vi "get information display strings.vi"(8 "error in":errorcluster, 11 "CEF_serializable node in":refnum<class "CEF_serializable node.lvclass">) -> (0 "error out":errorcluster, 1 "Data":string[](array[string]), 2 "Labels":string[](array[string]), 3 "CEF_serializable node out":refnum<class "CEF_serializable node.lvclass">)   [LabVIEW 2025, in "CEF.lvlib" / "CEF_serializable node.lvclass"]
doc: "Copyright 2017 National Instruments Corporation\n\nLicensed under the Apache License, Version 2.0 (the \"License\"); you may not use this file except in compliance with the License. You may obtain a copy of the License at http://www.apache.org/licenses/LICENSE-2.0\nUnless required by applicable law or agreed to in writing, software distributed under the License is distributed on an \"AS IS\" BASIS, WITHOUT WARRANTIES OR CONDITIONS OF ANY KIND, either express or implied. See the License for the specific language governing permissions and limitations under the License."
uses:
  CEF_serializable node.lvclass
  serializable configuration/CEF_serializable configuration.lvclass/CEF_serializable configuration.ctl
  <vilib>/Utility/LVClass/Get LV Class Name.vi
  error generator/CEF_error generator.vi
  serializable configuration/CEF_serializable configuration.lvclass
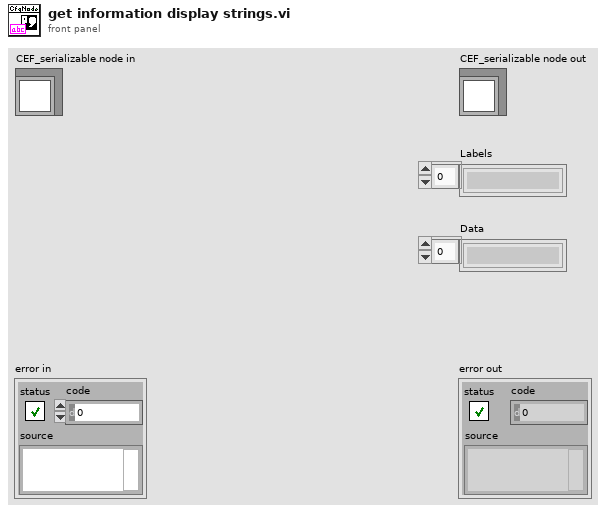
[diagram p1: front panel]
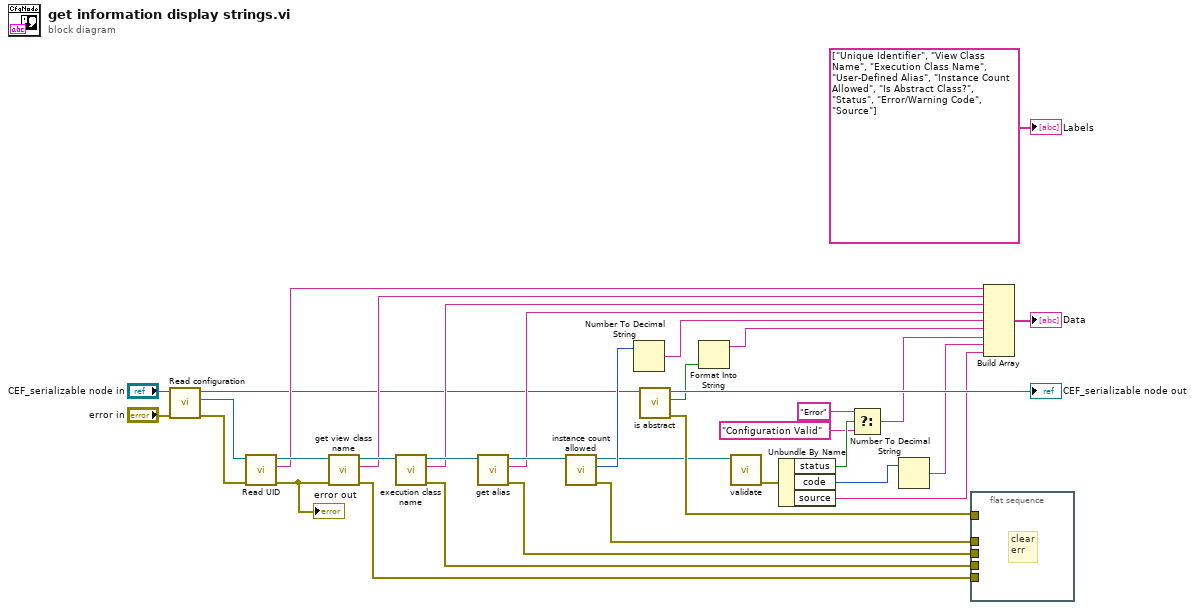
[diagram p0: block diagram]
diagram:
  n1 = call-dynamic "Read configuration.vi"("error in"="error in", "CEF_serializable node in"="CEF_serializable node in") -> ("error out"=w28:errorcluster, "CEF Configuration"=w13:refnum<class "CEF_serializable configuration.lvclass">, "CEF_serializable node out"=w6:refnum<class "CEF_serializable node.lvclass">)  [unwired: 7 in]
  n2 = call "Read UID.vi"("error in"=w28, "CEF_Configuration in"=w13) -> ("error out"=w19:errorcluster, "instance id"=w20:string, "CEF_Configuration out"=w32:refnum<class "CEF_serializable configuration.lvclass">)  [unwired: 7 in]
  "error out" <- w19
  n3 = call "get view class name.vi"("error in"=w19, "CEF_Configuration in"=w32) -> ("error out"=w18:errorcluster, "view class"=w21:string, "CEF_Configuration out"=w31:refnum<class "CEF_serializable configuration.lvclass">)  [unwired: 7 in]
  n4 = call-dynamic "execution class name.vi"("CEF_Configuration in"=w31) -> ("error out"=w17:errorcluster, "execution class"=w22:string, "CEF_Configuration out"=w30:refnum<class "CEF_serializable configuration.lvclass">)  [unwired: 8 in]
  n5 = call "get alias.vi"("CEF_Configuration in"=w30) -> ("error out"=w16:errorcluster, "alias"=w23:string, "CEF_Configuration out"=w29:refnum<class "CEF_serializable configuration.lvclass">)  [unwired: 8 in]
  n6 = call-dynamic "instance count allowed.vi"("CEF_Configuration in"=w29) -> ("error out"=w15:errorcluster, "instances allowed"=w25:i32, "CEF_Configuration out"=w7:refnum<class "CEF_serializable configuration.lvclass">)  [unwired: 8 in]
  n7 = Number To Decimal String(number=w25) -> (decimal integer string=w24:string)  [unwired: 1 in]
  n8 = call-dynamic "is abstract.vi"("CEF_serializable node in"=w6) -> ("error out"=w14:errorcluster, "abstract"=w5:bool, "CEF_serializable node out"=→"CEF_serializable node out":refnum<class "CEF_serializable node.lvclass">)  [unwired: 8 in]
  n9 = Format Into String(w5) -> (resulting string=w3:string)  [unwired: 3 in, 1 out]
  n10 = call-dynamic "validate.vi"("CEF_Configuration in"=w7) -> ("error out"=w12:errorcluster)  [unwired: 9 in, 1 out]
  n11 = Unbundle By Name(w12) -> ("status"=w11:bool, "code"=w9:i32, "source"=w10:string)
  n12 = Select(t="Error", s=w11, f="Configuration Valid") -> (s? t:f=w4:string)
  n13 = Number To Decimal String(number=w9) -> (decimal integer string=w8:string)  [unwired: 1 in]
  n14 = flat-sequence {
    tunnel: w18 -> [_]
    tunnel: w17 -> [_]
    tunnel: w16 -> [_]
    tunnel: w15 -> [_]
    tunnel: w14 -> [_]
    frame #0 {
      # "clear\nerr"
    }
  }
  n15 = Build Array(w20, w21, w22, w23, w24, w3, w4, w8, w10) -> (→"Data":string[])
  "Labels" <- string[] ["Unique Identifier", "View Class Name", "Execution Class Name", "User-Defined Alias", "Instance Count Allowed", "Is Abstract Class?", "Status", "Error/Warning Code", "Source"] ("Labels")
